vi "WPI_CANJaguar_ScheduleStatusUpdates.vi"(6 "Update Period (s)":dbl=0.1, 8 "error in (no error)":errorcluster, 9 "Status Channel Select":T1, 10 "Status Select":T2[](array[typedef]), 11 "CAN Jaguar Ref":T3={"DeviceStatus"={"status"=FALSE, "code"=0, "source"=""}, "Type"=enum."PWM", "PWM"={"PWM Channel"=enum."PWM 1", "DeadBand"={"Name"="", "maxPositivePwm"=0, "minPositivePwm"=0, "centerPwm"=0, "maxNegativePwm"=0, "minNegativePwm"=0, "angularRange"=0}}, "CAN"={"Device Number"=0, "SetOutput VI Ref"=variant(enum8{"Percent VBus", "Current", "Speed", "Position", "Voltage"} enum."Percent VBus"), "GetOutput VI Ref"=variant(refnum<k1> refnum), "Enable VI Ref"=variant(dbl 12.0), "Disable VI Ref"=variant(enum8{"Percent VBus", "Speed", "Position", "Slave", "Unchanged / Invalid", "Voltage Compensation", "Current", "Motion Profile"} enum."Percent VBus"), "Data"=variant}, "Invert"=FALSE}) -> (0 "error out":errorcluster, 3 "CAN Jaguar Ref Out":T3={"DeviceStatus"={"status"=FALSE, "code"=0, "source"=""}, "Type"=enum."PWM", "PWM"={"PWM Channel"=enum."PWM 1", "DeadBand"={"Name"="", "maxPositivePwm"=0, "minPositivePwm"=0, "centerPwm"=0, "maxNegativePwm"=0, "minNegativePwm"=0, "angularRange"=0}}, "CAN"={"Device Number"=0, "SetOutput VI Ref"=variant(enum8{"Percent VBus", "Current", "Speed", "Position", "Voltage"} enum."Percent VBus"), "GetOutput VI Ref"=variant(refnum<k1> refnum), "Enable VI Ref"=variant(dbl 12.0), "Disable VI Ref"=variant(enum8{"Percent VBus", "Speed", "Position", "Slave", "Unchanged / Invalid", "Voltage Compensation", "Current", "Motion Profile"} enum."Percent VBus"), "Data"=variant}, "Invert"=FALSE})   [LabVIEW 2016]
doc: "Schedule periodic status updates from a CAN Jaguar.\n\nThis VI allows you to specify which parts of the status you care about and how often you want to be updated. If used appropriately, this could reduce the bandwidth needed to get status by more than 50% because the request message is not sent for each update and multiple status values are packaged into a single message.\n\nThe periodic status messages can return 8 bytes of status data on each channel. Be sure that the status messages you select for each channel add up to 8 bytes or less. Output Voltage, Bus Voltage, Current, and Temperature are 2 bytes each. Position and Speed are 4 bytes each. Limit Switches and Faults are 1 byte each. Fault Counters are 8 bytes. Power Cycle is not supported.\n\nSticky Limit Switches, Faults, and Fault Counters are cleared by reading the respective status by calling <B>Get Status</B> VI with <B>Status Channel Select</B> set to <B>On Demand</B>.\n\nWire an empty <B>Status Select</B> array to disable periodic status updates for the channel.\n\nCall the <B>Get Status</B> VI with matching <B>Status Channel Select</B> to read the most recent values sent by the Jaguar."
uses:
  <vilib>/Rock Robotics/WPI/MotorControl/WPI_MotorControlDeviceRef.ctl
  <vilib>/Rock Robotics/WPI/MotorControl/WPI_MotorControlType.ctl
  <vilib>/Rock Robotics/SystemInterfaces/DIO/FPGA_DIOPWMChannel.ctl
  <vilib>/Rock Robotics/WPI/PWM/WPI_PWMDeadband.ctl
  <vilib>/Rock Robotics/WPI/ThirdParty/CanMotor/CAN Jaguar/SubVIs/WPI_CANJaguar_StatusSelect.ctl
  <vilib>/Rock Robotics/WPI/ThirdParty/CanMotor/CAN Jaguar/SubVIs/WPI_CANJaguar_StatusChannelSelect.ctl
  <vilib>/Rock Robotics/WPI/ThirdParty/CanMotor/CAN Jaguar/SubVIs/WPI_CAN_PeriodicStatusIDs.ctl
  <vilib>/Rock Robotics/WPI/ThirdParty/CanMotor/CAN Jaguar/SubVIs/WPI_CAN_MotorMessageIDs.ctl
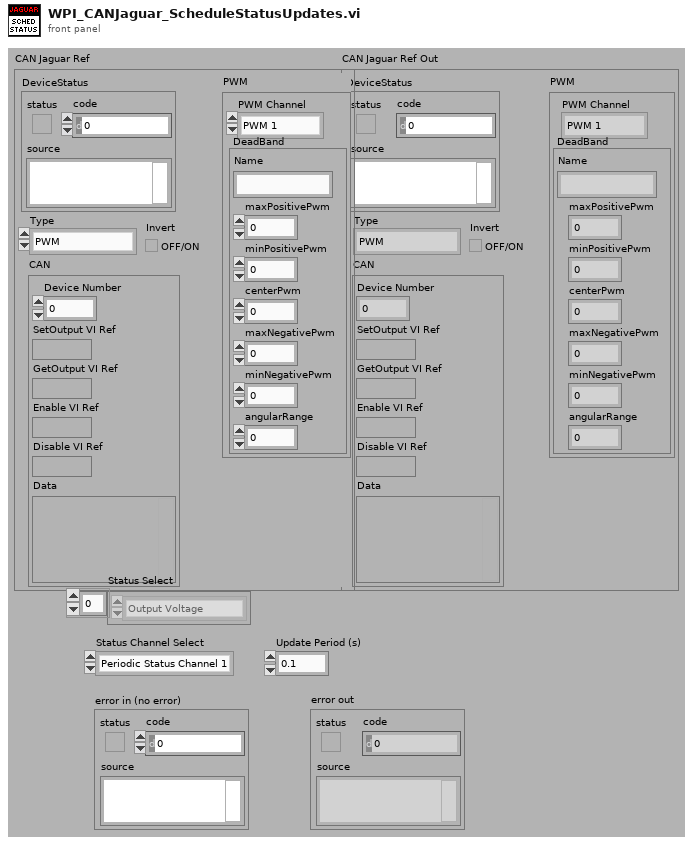
[diagram p1: front panel]
types:
  T1 = typedef "WPI_CANJaguar_StatusChannelSelect.ctl" = enum16{"Periodic Status Channel 1", "Periodic Status Channel 2", "Periodic Status Channel 3", "Periodic Status Channel 4", "On Demand Status"}
  T2 = typedef "WPI_CANJaguar_StatusSelect.ctl" = enum16{"Output Percent VBus", "Output Voltage", "Bus Voltage", "Current", "Temperature", "Position", "Speed", "Limit Switches", "Faults", "Fault Counters", "Power Cycle"}
  T3 = typedef "WPI_MotorControlDeviceRef.ctl" = cluster{"DeviceStatus":errorcluster, "Type":T4, "PWM":cluster{"PWM Channel":T5, "DeadBand":T6}, "CAN":cluster{"Device Number":u8, "SetOutput VI Ref":variant, "GetOutput VI Ref":variant, "Enable VI Ref":variant, "Disable VI Ref":variant, "Data":variant}, "Invert":bool}
  T4 = typedef "WPI_MotorControlType.ctl" = enum16{"PWM", "CAN"}
  T5 = typedef "FPGA_DIOPWMChannel.ctl" = enum8{"PWM 0", "PWM 1", "PWM 2", "PWM 3", "PWM 4", "PWM 5", "PWM 6", "PWM 7", "PWM 8", "PWM 9", "PWM MXP 0", "PWM MXP 1", "PWM MXP 2", "PWM MXP 3", "PWM MXP 4", "PWM MXP 5", "PWM MXP 6", "PWM MXP 7", "PWM MXP 8", "PWM MXP 9", "Invalid"}
  T6 = typedef "WPI_PWMDeadband.ctl" = cluster{"Name":string, "maxPositivePwm":i32, "minPositivePwm":i32, "centerPwm":i32, "maxNegativePwm":i32, "minNegativePwm":i32, "angularRange":u16}
  T7 = typedef "WPI_CAN_PeriodicStatusIDs.ctl" = enum16{"Disabled", "Percent VBus Out (Byte 0)", "Percent VBus Out (Byte 1)", "VBus (Byte 0)", "VBus (Byte 1)", "Current (Byte 0)", "Current (Byte 1)", "Temperature (Byte 0)", "Temperature (Byte 1)", "Position (Byte 0)", "Position (Byte 1)", "Position (Byte 2)", "Position (Byte 3)", "Speed (Byte 0)", "Speed (Byte 1)", "Speed (Byte 2)", "Speed (Byte 3)", "Limit Switches (No Clear)", "Limit Switches (Clear)", "Faults", "Sticky Faults (No Clear)", "Sticky Faults (Clear)", "Volts Out (Byte 0)", "Volts Out (Byte 1)", "Current Fault Counter", "Temperature Fault Counter", "VBus Fault Counter", "Gate Driver Fault Counter", "Comm Fault Counter", "CANSTS", "CANERR (Byte 0)", "CANERR (Byte 1)", "Power Cycle"}
  T8 = enum16{"big-endian, network order", "native, host order", "little-endian"}
  T9 = typedef "WPI_CAN_MotorMessageIDs.ctl" = u32
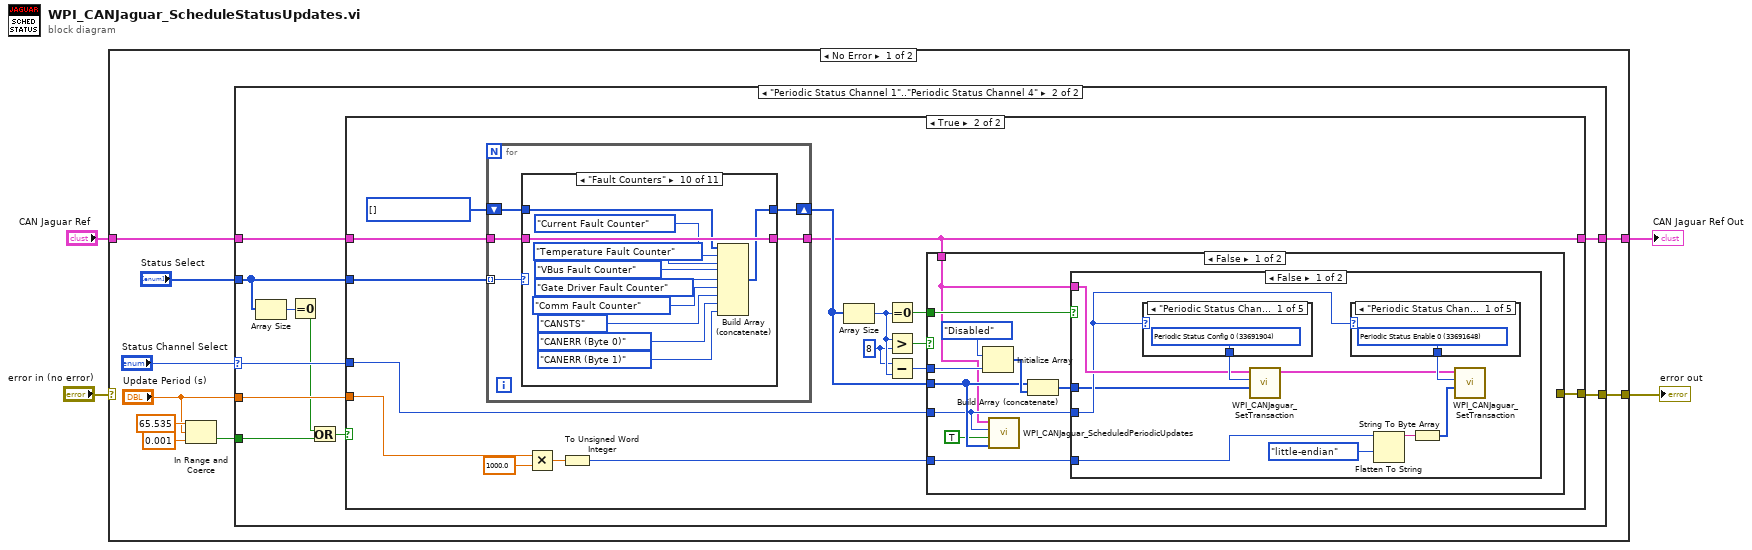
[diagram p0: block diagram]
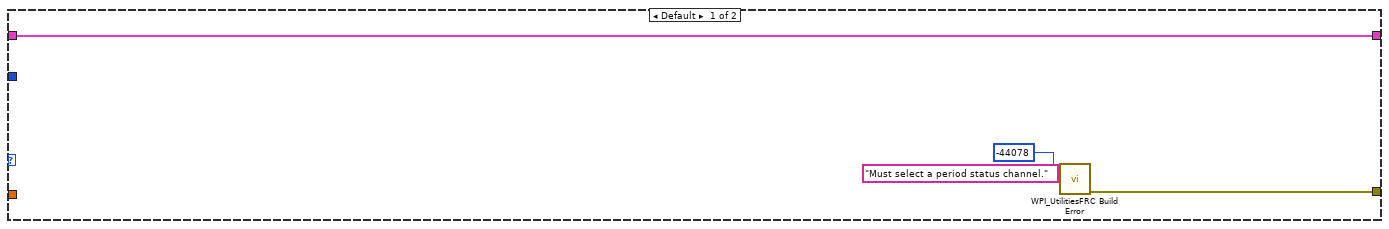
[diagram p2: hidden frame]
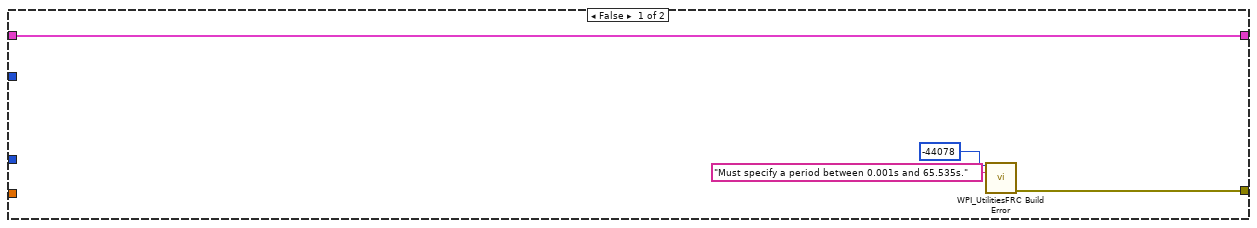
[diagram p3: hidden frame]
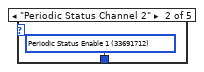
[diagram p4: hidden frame]
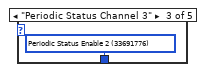
[diagram p5: hidden frame]
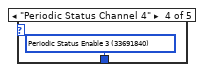
[diagram p6: hidden frame]
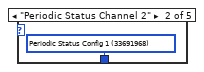
[diagram p8: hidden frame]
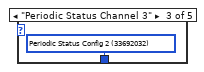
[diagram p9: hidden frame]
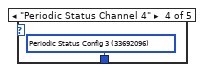
[diagram p10: hidden frame]
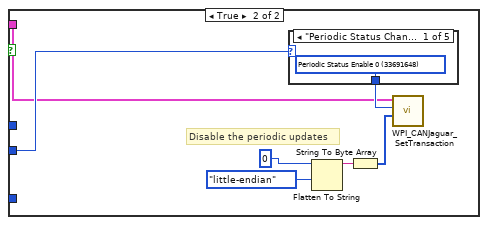
[diagram p12: hidden frame]
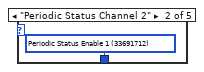
[diagram p13: hidden frame]
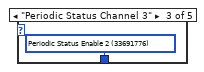
[diagram p14: hidden frame]
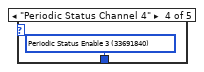
[diagram p15: hidden frame]
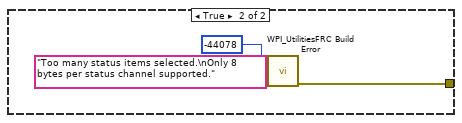
[diagram p17: hidden frame]
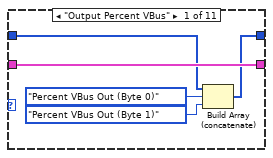
[diagram p18: hidden frame]
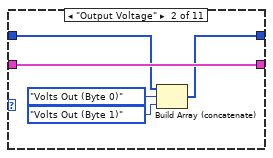
[diagram p19: hidden frame]
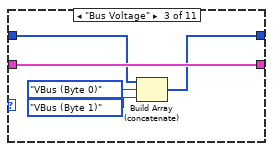
[diagram p20: hidden frame]
diagram:
  n1 = case shown="No Error" "error in (no error)" {
    selector: "error in (no error)" -> [_ w156]
    tunnel: [w11 w155] -> w4
    tunnel: "CAN Jaguar Ref" -> [w13 w155]
    tunnel: [w12 w156] -> w2
    frame No Error {
      n2 = In Range and Coerce(upper limit=65.535, x="Update Period (s)", lower limit=0.001) -> (In Range?=w9:bool)  [unwired: 1 out]
      n3 = case shown="\"Periodic Status Channel 1\"..\"Periodic Status Channel 4\"" "Status Channel Select" {
        selector: "Status Channel Select" -> [_ w24]
        tunnel: w13 -> [w14 w27]
        tunnel: [w15 w26] -> w12
        tunnel: [w14 w25] -> w11
        tunnel: w9 -> [_ w20]
        tunnel: "Update Period (s)" -> [_ w23]
        tunnel: "Status Select" -> [_ w21]
        frame Default {
          n4 = call <vilib>:"WPI_UtilitiesFRC Build Error.vi"("error code"=-44078, "extra error text"="Must select a period status channel.") -> ("error out"=w15:errorcluster)  [unwired: 3 in, 10 out]
        }
        frame "Periodic Status Channel 1".."Periodic Status Channel 4" {
          n5 = Array Size(array=w21) -> (size(s)=w22:i32)
          n6 = Equal To 0?(x=w22) -> (x = 0?=w18:bool)
          n7 = Or(x=w18, y=w20) -> (x .or. y?=w19:bool)
          n8 = case shown="True" w19 {
            tunnel: w27 -> [w28 w47]
            tunnel: [w29 w44] -> w26
            tunnel: [w28 w42] -> w25
            tunnel: w24 -> [_ w41]
            tunnel: w23 -> [_ w40]
            tunnel: w21 -> [_ w32]
            frame False {
              n9 = call <vilib>:"WPI_UtilitiesFRC Build Error.vi"("error code"=-44078, "extra error text"="Must specify a period between 0.001s and 65.535s.") -> ("error out"=w29:errorcluster)  [unwired: 3 in, 10 out]
            }
            frame True {
              w34 = 8 ("y")
              w46 = T7[] [] items=["Disabled", "Percent VBus Out (Byte 0)", "Percent VBus Out (Byte 1)", "VBus (Byte 0)", "VBus (Byte 1)", "Current (Byte 0)", "Current (Byte 1)", "Temperature (Byte 0)", "Temperature (Byte 1)", "Position (Byte 0)", "Position (Byte 1)", "Position (Byte 2)", "Position (Byte 3)", "Speed (Byte 0)", "Speed (Byte 1)", "Speed (Byte 2)", "Speed (Byte 3)", "Limit Switches (No Clear)", "Limit Switches (Clear)", "Faults", "Sticky Faults (No Clear)", "Sticky Faults (Clear)", "Volts Out (Byte 0)", "Volts Out (Byte 1)", "Current Fault Counter", "Temperature Fault Counter", "VBus Fault Counter", "Gate Driver Fault Counter", "Comm Fault Counter", "CANSTS", "CANERR (Byte 0)", "CANERR (Byte 1)", "Power Cycle"]
              n10 = for {
                tunnel: w32 -> [w94] mode=indexing
                tunnel: w47 -> [w93]
                tunnel: [w92] -> w42
                shift-right: [w90] -> w43
                shift-left: w46 -> [w91]
                n11 = case shown="\"Fault Counters\"" w94 {
                  tunnel: w93 -> [w99 w104 w109 w114 w119 w126 w133 w137 w141 w152 w154]
                  tunnel: [w99 w104 w109 w114 w119 w126 w133 w137 w141 w152 w154] -> w92
                  tunnel: w91 -> [w98 w103 w108 w113 w118 w125 w131 w136 w140 w151 w153]
                  tunnel: [w97 w102 w105 w112 w117 w124 w130 w135 w139 w150 w153] -> w90
                  frame "Output Percent VBus" {
                    n12 = Build Array (concatenate)(w98, WPI_CAN_PeriodicStatusIDs."Percent VBus Out (Byte 0)" ("Periodic Status IDs"), WPI_CAN_PeriodicStatusIDs."Percent VBus Out (Byte 1)" ("Periodic Status IDs")) -> (w97:T7[])
                  }
                  frame "Output Voltage" {
                    n13 = Build Array (concatenate)(w103, WPI_CAN_PeriodicStatusIDs."Volts Out (Byte 0)" ("Periodic Status IDs"), WPI_CAN_PeriodicStatusIDs."Volts Out (Byte 1)" ("Periodic Status IDs")) -> (w102:T7[])
                  }
                  frame "Bus Voltage" {
                    n14 = Build Array (concatenate)(w108, WPI_CAN_PeriodicStatusIDs."VBus (Byte 0)" ("Periodic Status IDs"), WPI_CAN_PeriodicStatusIDs."VBus (Byte 1)" ("Periodic Status IDs")) -> (w105:T7[])
                  }
                  frame "Current" {
                    n15 = Build Array (concatenate)(w113, WPI_CAN_PeriodicStatusIDs."Current (Byte 0)" ("Periodic Status IDs"), WPI_CAN_PeriodicStatusIDs."Current (Byte 1)" ("Periodic Status IDs")) -> (w112:T7[])
                  }
                  frame "Temperature" {
                    n16 = Build Array (concatenate)(w118, WPI_CAN_PeriodicStatusIDs."Temperature (Byte 0)" ("Periodic Status IDs"), WPI_CAN_PeriodicStatusIDs."Temperature (Byte 1)" ("Periodic Status IDs")) -> (w117:T7[])
                  }
                  frame "Position" {
                    n17 = Build Array (concatenate)(w125, WPI_CAN_PeriodicStatusIDs."Position (Byte 0)" ("Periodic Status IDs"), WPI_CAN_PeriodicStatusIDs."Position (Byte 1)" ("Periodic Status IDs"), WPI_CAN_PeriodicStatusIDs."Position (Byte 2)" ("Periodic Status IDs"), WPI_CAN_PeriodicStatusIDs."Position (Byte 3)" ("Periodic Status IDs")) -> (w124:T7[])
                  }
                  frame "Speed" {
                    n18 = Build Array (concatenate)(w131, WPI_CAN_PeriodicStatusIDs."Speed (Byte 0)" ("Periodic Status IDs"), WPI_CAN_PeriodicStatusIDs."Speed (Byte 1)" ("Periodic Status IDs"), WPI_CAN_PeriodicStatusIDs."Speed (Byte 2)" ("Periodic Status IDs"), WPI_CAN_PeriodicStatusIDs."Speed (Byte 3)" ("Periodic Status IDs")) -> (w130:T7[])
                  }
                  frame "Limit Switches" {
                    n19 = Build Array (concatenate)(w136, WPI_CAN_PeriodicStatusIDs."Limit Switches (No Clear)" ("Periodic Status IDs")) -> (w135:T7[])
                  }
                  frame "Faults" {
                    n20 = Build Array (concatenate)(w140, WPI_CAN_PeriodicStatusIDs."Sticky Faults (No Clear)" ("Periodic Status IDs")) -> (w139:T7[])
                  }
                  frame "Fault Counters" {
                    n21 = Build Array (concatenate)(w151, WPI_CAN_PeriodicStatusIDs."Current Fault Counter" ("Periodic Status IDs"), WPI_CAN_PeriodicStatusIDs."Temperature Fault Counter" ("Periodic Status IDs"), WPI_CAN_PeriodicStatusIDs."VBus Fault Counter" ("Periodic Status IDs"), WPI_CAN_PeriodicStatusIDs."Gate Driver Fault Counter" ("Periodic Status IDs"), WPI_CAN_PeriodicStatusIDs."Comm Fault Counter" ("Periodic Status IDs"), WPI_CAN_PeriodicStatusIDs."CANSTS" ("Periodic Status IDs"), WPI_CAN_PeriodicStatusIDs."CANERR (Byte 0)" ("Periodic Status IDs"), WPI_CAN_PeriodicStatusIDs."CANERR (Byte 1)" ("Periodic Status IDs")) -> (w150:T7[])
                  }
                  frame "Power Cycle" {
                  }
                }
              }
              n22 = Multiply(x=w40, y=1000.0) -> (x*y=w38:dbl)
              n23 = To Unsigned Word Integer(number=w38) -> (unsigned 16bit integer=w37:u16)
              n24 = Array Size(array=w43) -> (size(s)=w35:i32)
              n25 = Equal To 0?(x=w35) -> (x = 0?=w36:bool)
              n26 = Greater?(x=w35, y=w34) -> (0:w45:bool)
              n27 = Subtract(x=w34, y=w35) -> (x-y=w33:i32)
              n28 = case shown="False" w45 {
                tunnel: [_ w87] -> w44
                tunnel: w43 -> [w51 _]
                tunnel: w42 -> [w48 _]
                tunnel: w41 -> [w49 _]
                tunnel: w37 -> [w57 _]
                tunnel: w36 -> [w56 _]
                tunnel: w33 -> [w55 _]
                frame False {
                  n29 = Initialize Array(WPI_CAN_PeriodicStatusIDs."Disabled" ("Periodic Status IDs"), w55) -> (w52:T7[])
                  n30 = call <vilib>:"WPI_CANJaguar_ScheduledPeriodicUpdates.vi"("Fields In"=w51, "Update"=TRUE, "Status Channel Select"=w49, "CAN Jaguar Ref"=w48) -> ()  [unwired: 7 in, 1 out]
                  n31 = Build Array (concatenate)(w51, w52) -> (w53:T7[])
                  n32 = case shown="False" w56 {
                    tunnel: w48 -> [w65 w76]
                    tunnel: w57 -> [w60 _]
                    tunnel: w49 -> [w59 w77]
                    tunnel: w53 -> [w58 _]
                    frame False {
                      n33 = case shown="\"Periodic Status Channel 1\"" w59 {
                        tunnel: [w72 w73 w74 w75 _] -> w67
                        frame "Periodic Status Channel 1" {
                          w72 = T9 33691904 items=["Volt Enable"=33685504, "Volt Disable"=33685568, "Volt Set"=33685632, "Volt Set Ramp"=33685696, "Volt Set No Ack"=33686080, "Speed Enable"=33686528, "Speed Disable"=33686592, "Speed Set"=33686656, "Speed P"=33686720, "Speed I"=33686784, "Speed D"=33686848, "Speed Ref"=33686912, "Speed Set No Ack"=33687232, "Volt Comp Enable"=33687552, "Volt Comp Disable"=33687616, "Volt Comp Set"=33687680, "Volt Comp In Ramp"=33687744, "Volt Comp Comp Ramp"=33687808, "Volt Comp Set No Ack"=33688128, "Position Enable"=33688576, "Position Disable"=33688640, "Position Set"=33688704, "Position P"=33688768, "Position I"=33688832, "Position D"=33688896, "Position Ref"=33688960, "Position Set No Ack"=33689280, "Current Enable"=33689600, "Current Disable"=33689664, "Current Set"=33689728, "Current P"=33689792, "Current I"=33689856, "Current D"=33689920, "Current Set No Ack"=33690240, "Status Percent VBus"=33690624, "Status VBus"=33690688, "Status Current"=33690752, "Status Temp"=33690816, "Status Position"=33690880, "Status Speed"=33690944, "Status Limit"=33691008, "Status Fault"=33691072, "Status Power"=33691136, "Status Control Mode"=33691200, "Status VOut"=33691264, "Status Sticky Fault"=33691328, "Status Fault Count"=33691392, "Periodic Status Enable 0"=33691648, "Periodic Status Enable 1"=33691712, "Periodic Status Enable 2"=33691776, "Periodic Status Enable 3"=33691840, "Periodic Status Config 0"=33691904, "Periodic Status Config 1"=33691968, "Periodic Status Config 2"=33692032, "Periodic Status Config 3"=33692096, "Periodic Status Data 0"=33692160, "Periodic Status Data 1"=33692224, "Periodic Status Data 2"=33692288, "Periodic Status Data 3"=33692352, "Config Num Brushes"=33692672, "Config Encoder Lines"=33692736, "Config Pot Turns"=33692800, "Config Brake Coast"=33692864, "Config Limit Mode"=33692928, "Config Limit Fwd"=33692992, "Config Limit Rev"=33693056, "Config Max VOut"=33693120, "Config Fault Time"=33693184, "Motor Ack"=33693696] ("CAN Motor Message IDs")
                        }
                        frame "Periodic Status Channel 2" {
                          w73 = T9 33691968 items=["Volt Enable"=33685504, "Volt Disable"=33685568, "Volt Set"=33685632, "Volt Set Ramp"=33685696, "Volt Set No Ack"=33686080, "Speed Enable"=33686528, "Speed Disable"=33686592, "Speed Set"=33686656, "Speed P"=33686720, "Speed I"=33686784, "Speed D"=33686848, "Speed Ref"=33686912, "Speed Set No Ack"=33687232, "Volt Comp Enable"=33687552, "Volt Comp Disable"=33687616, "Volt Comp Set"=33687680, "Volt Comp In Ramp"=33687744, "Volt Comp Comp Ramp"=33687808, "Volt Comp Set No Ack"=33688128, "Position Enable"=33688576, "Position Disable"=33688640, "Position Set"=33688704, "Position P"=33688768, "Position I"=33688832, "Position D"=33688896, "Position Ref"=33688960, "Position Set No Ack"=33689280, "Current Enable"=33689600, "Current Disable"=33689664, "Current Set"=33689728, "Current P"=33689792, "Current I"=33689856, "Current D"=33689920, "Current Set No Ack"=33690240, "Status Percent VBus"=33690624, "Status VBus"=33690688, "Status Current"=33690752, "Status Temp"=33690816, "Status Position"=33690880, "Status Speed"=33690944, "Status Limit"=33691008, "Status Fault"=33691072, "Status Power"=33691136, "Status Control Mode"=33691200, "Status VOut"=33691264, "Status Sticky Fault"=33691328, "Status Fault Count"=33691392, "Periodic Status Enable 0"=33691648, "Periodic Status Enable 1"=33691712, "Periodic Status Enable 2"=33691776, "Periodic Status Enable 3"=33691840, "Periodic Status Config 0"=33691904, "Periodic Status Config 1"=33691968, "Periodic Status Config 2"=33692032, "Periodic Status Config 3"=33692096, "Periodic Status Data 0"=33692160, "Periodic Status Data 1"=33692224, "Periodic Status Data 2"=33692288, "Periodic Status Data 3"=33692352, "Config Num Brushes"=33692672, "Config Encoder Lines"=33692736, "Config Pot Turns"=33692800, "Config Brake Coast"=33692864, "Config Limit Mode"=33692928, "Config Limit Fwd"=33692992, "Config Limit Rev"=33693056, "Config Max VOut"=33693120, "Config Fault Time"=33693184, "Motor Ack"=33693696] ("CAN Motor Message IDs")
                        }
                        frame "Periodic Status Channel 3" {
                          w74 = T9 33692032 items=["Volt Enable"=33685504, "Volt Disable"=33685568, "Volt Set"=33685632, "Volt Set Ramp"=33685696, "Volt Set No Ack"=33686080, "Speed Enable"=33686528, "Speed Disable"=33686592, "Speed Set"=33686656, "Speed P"=33686720, "Speed I"=33686784, "Speed D"=33686848, "Speed Ref"=33686912, "Speed Set No Ack"=33687232, "Volt Comp Enable"=33687552, "Volt Comp Disable"=33687616, "Volt Comp Set"=33687680, "Volt Comp In Ramp"=33687744, "Volt Comp Comp Ramp"=33687808, "Volt Comp Set No Ack"=33688128, "Position Enable"=33688576, "Position Disable"=33688640, "Position Set"=33688704, "Position P"=33688768, "Position I"=33688832, "Position D"=33688896, "Position Ref"=33688960, "Position Set No Ack"=33689280, "Current Enable"=33689600, "Current Disable"=33689664, "Current Set"=33689728, "Current P"=33689792, "Current I"=33689856, "Current D"=33689920, "Current Set No Ack"=33690240, "Status Percent VBus"=33690624, "Status VBus"=33690688, "Status Current"=33690752, "Status Temp"=33690816, "Status Position"=33690880, "Status Speed"=33690944, "Status Limit"=33691008, "Status Fault"=33691072, "Status Power"=33691136, "Status Control Mode"=33691200, "Status VOut"=33691264, "Status Sticky Fault"=33691328, "Status Fault Count"=33691392, "Periodic Status Enable 0"=33691648, "Periodic Status Enable 1"=33691712, "Periodic Status Enable 2"=33691776, "Periodic Status Enable 3"=33691840, "Periodic Status Config 0"=33691904, "Periodic Status Config 1"=33691968, "Periodic Status Config 2"=33692032, "Periodic Status Config 3"=33692096, "Periodic Status Data 0"=33692160, "Periodic Status Data 1"=33692224, "Periodic Status Data 2"=33692288, "Periodic Status Data 3"=33692352, "Config Num Brushes"=33692672, "Config Encoder Lines"=33692736, "Config Pot Turns"=33692800, "Config Brake Coast"=33692864, "Config Limit Mode"=33692928, "Config Limit Fwd"=33692992, "Config Limit Rev"=33693056, "Config Max VOut"=33693120, "Config Fault Time"=33693184, "Motor Ack"=33693696] ("CAN Motor Message IDs")
                        }
                        frame "Periodic Status Channel 4" {
                          w75 = T9 33692096 items=["Volt Enable"=33685504, "Volt Disable"=33685568, "Volt Set"=33685632, "Volt Set Ramp"=33685696, "Volt Set No Ack"=33686080, "Speed Enable"=33686528, "Speed Disable"=33686592, "Speed Set"=33686656, "Speed P"=33686720, "Speed I"=33686784, "Speed D"=33686848, "Speed Ref"=33686912, "Speed Set No Ack"=33687232, "Volt Comp Enable"=33687552, "Volt Comp Disable"=33687616, "Volt Comp Set"=33687680, "Volt Comp In Ramp"=33687744, "Volt Comp Comp Ramp"=33687808, "Volt Comp Set No Ack"=33688128, "Position Enable"=33688576, "Position Disable"=33688640, "Position Set"=33688704, "Position P"=33688768, "Position I"=33688832, "Position D"=33688896, "Position Ref"=33688960, "Position Set No Ack"=33689280, "Current Enable"=33689600, "Current Disable"=33689664, "Current Set"=33689728, "Current P"=33689792, "Current I"=33689856, "Current D"=33689920, "Current Set No Ack"=33690240, "Status Percent VBus"=33690624, "Status VBus"=33690688, "Status Current"=33690752, "Status Temp"=33690816, "Status Position"=33690880, "Status Speed"=33690944, "Status Limit"=33691008, "Status Fault"=33691072, "Status Power"=33691136, "Status Control Mode"=33691200, "Status VOut"=33691264, "Status Sticky Fault"=33691328, "Status Fault Count"=33691392, "Periodic Status Enable 0"=33691648, "Periodic Status Enable 1"=33691712, "Periodic Status Enable 2"=33691776, "Periodic Status Enable 3"=33691840, "Periodic Status Config 0"=33691904, "Periodic Status Config 1"=33691968, "Periodic Status Config 2"=33692032, "Periodic Status Config 3"=33692096, "Periodic Status Data 0"=33692160, "Periodic Status Data 1"=33692224, "Periodic Status Data 2"=33692288, "Periodic Status Data 3"=33692352, "Config Num Brushes"=33692672, "Config Encoder Lines"=33692736, "Config Pot Turns"=33692800, "Config Brake Coast"=33692864, "Config Limit Mode"=33692928, "Config Limit Fwd"=33692992, "Config Limit Rev"=33693056, "Config Max VOut"=33693120, "Config Fault Time"=33693184, "Motor Ack"=33693696] ("CAN Motor Message IDs")
                        }
                        frame Default {
                          # "This won't happen"
                        }
                      }
                      n34 = call <vilib>:"WPI_CANJaguar_SetTransaction.vi"("Data"=w58, "Message ID"=w67, "CAN Jaguar Ref"=w65) -> ("CAN Jaguar Ref Out"=w64:T3)  [unwired: 1 in, 7 out]
                      n35 = case shown="\"Periodic Status Channel 1\"" w59 {
                        tunnel: [w68 w69 w70 w71 _] -> w66
                        frame "Periodic Status Channel 1" {
                          w68 = T9 33691648 items=["Volt Enable"=33685504, "Volt Disable"=33685568, "Volt Set"=33685632, "Volt Set Ramp"=33685696, "Volt Set No Ack"=33686080, "Speed Enable"=33686528, "Speed Disable"=33686592, "Speed Set"=33686656, "Speed P"=33686720, "Speed I"=33686784, "Speed D"=33686848, "Speed Ref"=33686912, "Speed Set No Ack"=33687232, "Volt Comp Enable"=33687552, "Volt Comp Disable"=33687616, "Volt Comp Set"=33687680, "Volt Comp In Ramp"=33687744, "Volt Comp Comp Ramp"=33687808, "Volt Comp Set No Ack"=33688128, "Position Enable"=33688576, "Position Disable"=33688640, "Position Set"=33688704, "Position P"=33688768, "Position I"=33688832, "Position D"=33688896, "Position Ref"=33688960, "Position Set No Ack"=33689280, "Current Enable"=33689600, "Current Disable"=33689664, "Current Set"=33689728, "Current P"=33689792, "Current I"=33689856, "Current D"=33689920, "Current Set No Ack"=33690240, "Status Percent VBus"=33690624, "Status VBus"=33690688, "Status Current"=33690752, "Status Temp"=33690816, "Status Position"=33690880, "Status Speed"=33690944, "Status Limit"=33691008, "Status Fault"=33691072, "Status Power"=33691136, "Status Control Mode"=33691200, "Status VOut"=33691264, "Status Sticky Fault"=33691328, "Status Fault Count"=33691392, "Periodic Status Enable 0"=33691648, "Periodic Status Enable 1"=33691712, "Periodic Status Enable 2"=33691776, "Periodic Status Enable 3"=33691840, "Periodic Status Config 0"=33691904, "Periodic Status Config 1"=33691968, "Periodic Status Config 2"=33692032, "Periodic Status Config 3"=33692096, "Periodic Status Data 0"=33692160, "Periodic Status Data 1"=33692224, "Periodic Status Data 2"=33692288, "Periodic Status Data 3"=33692352, "Config Num Brushes"=33692672, "Config Encoder Lines"=33692736, "Config Pot Turns"=33692800, "Config Brake Coast"=33692864, "Config Limit Mode"=33692928, "Config Limit Fwd"=33692992, "Config Limit Rev"=33693056, "Config Max VOut"=33693120, "Config Fault Time"=33693184, "Motor Ack"=33693696] ("CAN Motor Message IDs")
                        }
                        frame "Periodic Status Channel 2" {
                          w69 = T9 33691712 items=["Volt Enable"=33685504, "Volt Disable"=33685568, "Volt Set"=33685632, "Volt Set Ramp"=33685696, "Volt Set No Ack"=33686080, "Speed Enable"=33686528, "Speed Disable"=33686592, "Speed Set"=33686656, "Speed P"=33686720, "Speed I"=33686784, "Speed D"=33686848, "Speed Ref"=33686912, "Speed Set No Ack"=33687232, "Volt Comp Enable"=33687552, "Volt Comp Disable"=33687616, "Volt Comp Set"=33687680, "Volt Comp In Ramp"=33687744, "Volt Comp Comp Ramp"=33687808, "Volt Comp Set No Ack"=33688128, "Position Enable"=33688576, "Position Disable"=33688640, "Position Set"=33688704, "Position P"=33688768, "Position I"=33688832, "Position D"=33688896, "Position Ref"=33688960, "Position Set No Ack"=33689280, "Current Enable"=33689600, "Current Disable"=33689664, "Current Set"=33689728, "Current P"=33689792, "Current I"=33689856, "Current D"=33689920, "Current Set No Ack"=33690240, "Status Percent VBus"=33690624, "Status VBus"=33690688, "Status Current"=33690752, "Status Temp"=33690816, "Status Position"=33690880, "Status Speed"=33690944, "Status Limit"=33691008, "Status Fault"=33691072, "Status Power"=33691136, "Status Control Mode"=33691200, "Status VOut"=33691264, "Status Sticky Fault"=33691328, "Status Fault Count"=33691392, "Periodic Status Enable 0"=33691648, "Periodic Status Enable 1"=33691712, "Periodic Status Enable 2"=33691776, "Periodic Status Enable 3"=33691840, "Periodic Status Config 0"=33691904, "Periodic Status Config 1"=33691968, "Periodic Status Config 2"=33692032, "Periodic Status Config 3"=33692096, "Periodic Status Data 0"=33692160, "Periodic Status Data 1"=33692224, "Periodic Status Data 2"=33692288, "Periodic Status Data 3"=33692352, "Config Num Brushes"=33692672, "Config Encoder Lines"=33692736, "Config Pot Turns"=33692800, "Config Brake Coast"=33692864, "Config Limit Mode"=33692928, "Config Limit Fwd"=33692992, "Config Limit Rev"=33693056, "Config Max VOut"=33693120, "Config Fault Time"=33693184, "Motor Ack"=33693696] ("CAN Motor Message IDs")
                        }
                        frame "Periodic Status Channel 3" {
                          w70 = T9 33691776 items=["Volt Enable"=33685504, "Volt Disable"=33685568, "Volt Set"=33685632, "Volt Set Ramp"=33685696, "Volt Set No Ack"=33686080, "Speed Enable"=33686528, "Speed Disable"=33686592, "Speed Set"=33686656, "Speed P"=33686720, "Speed I"=33686784, "Speed D"=33686848, "Speed Ref"=33686912, "Speed Set No Ack"=33687232, "Volt Comp Enable"=33687552, "Volt Comp Disable"=33687616, "Volt Comp Set"=33687680, "Volt Comp In Ramp"=33687744, "Volt Comp Comp Ramp"=33687808, "Volt Comp Set No Ack"=33688128, "Position Enable"=33688576, "Position Disable"=33688640, "Position Set"=33688704, "Position P"=33688768, "Position I"=33688832, "Position D"=33688896, "Position Ref"=33688960, "Position Set No Ack"=33689280, "Current Enable"=33689600, "Current Disable"=33689664, "Current Set"=33689728, "Current P"=33689792, "Current I"=33689856, "Current D"=33689920, "Current Set No Ack"=33690240, "Status Percent VBus"=33690624, "Status VBus"=33690688, "Status Current"=33690752, "Status Temp"=33690816, "Status Position"=33690880, "Status Speed"=33690944, "Status Limit"=33691008, "Status Fault"=33691072, "Status Power"=33691136, "Status Control Mode"=33691200, "Status VOut"=33691264, "Status Sticky Fault"=33691328, "Status Fault Count"=33691392, "Periodic Status Enable 0"=33691648, "Periodic Status Enable 1"=33691712, "Periodic Status Enable 2"=33691776, "Periodic Status Enable 3"=33691840, "Periodic Status Config 0"=33691904, "Periodic Status Config 1"=33691968, "Periodic Status Config 2"=33692032, "Periodic Status Config 3"=33692096, "Periodic Status Data 0"=33692160, "Periodic Status Data 1"=33692224, "Periodic Status Data 2"=33692288, "Periodic Status Data 3"=33692352, "Config Num Brushes"=33692672, "Config Encoder Lines"=33692736, "Config Pot Turns"=33692800, "Config Brake Coast"=33692864, "Config Limit Mode"=33692928, "Config Limit Fwd"=33692992, "Config Limit Rev"=33693056, "Config Max VOut"=33693120, "Config Fault Time"=33693184, "Motor Ack"=33693696] ("CAN Motor Message IDs")
                        }
                        frame "Periodic Status Channel 4" {
                          w71 = T9 33691840 items=["Volt Enable"=33685504, "Volt Disable"=33685568, "Volt Set"=33685632, "Volt Set Ramp"=33685696, "Volt Set No Ack"=33686080, "Speed Enable"=33686528, "Speed Disable"=33686592, "Speed Set"=33686656, "Speed P"=33686720, "Speed I"=33686784, "Speed D"=33686848, "Speed Ref"=33686912, "Speed Set No Ack"=33687232, "Volt Comp Enable"=33687552, "Volt Comp Disable"=33687616, "Volt Comp Set"=33687680, "Volt Comp In Ramp"=33687744, "Volt Comp Comp Ramp"=33687808, "Volt Comp Set No Ack"=33688128, "Position Enable"=33688576, "Position Disable"=33688640, "Position Set"=33688704, "Position P"=33688768, "Position I"=33688832, "Position D"=33688896, "Position Ref"=33688960, "Position Set No Ack"=33689280, "Current Enable"=33689600, "Current Disable"=33689664, "Current Set"=33689728, "Current P"=33689792, "Current I"=33689856, "Current D"=33689920, "Current Set No Ack"=33690240, "Status Percent VBus"=33690624, "Status VBus"=33690688, "Status Current"=33690752, "Status Temp"=33690816, "Status Position"=33690880, "Status Speed"=33690944, "Status Limit"=33691008, "Status Fault"=33691072, "Status Power"=33691136, "Status Control Mode"=33691200, "Status VOut"=33691264, "Status Sticky Fault"=33691328, "Status Fault Count"=33691392, "Periodic Status Enable 0"=33691648, "Periodic Status Enable 1"=33691712, "Periodic Status Enable 2"=33691776, "Periodic Status Enable 3"=33691840, "Periodic Status Config 0"=33691904, "Periodic Status Config 1"=33691968, "Periodic Status Config 2"=33692032, "Periodic Status Config 3"=33692096, "Periodic Status Data 0"=33692160, "Periodic Status Data 1"=33692224, "Periodic Status Data 2"=33692288, "Periodic Status Data 3"=33692352, "Config Num Brushes"=33692672, "Config Encoder Lines"=33692736, "Config Pot Turns"=33692800, "Config Brake Coast"=33692864, "Config Limit Mode"=33692928, "Config Limit Fwd"=33692992, "Config Limit Rev"=33693056, "Config Max VOut"=33693120, "Config Fault Time"=33693184, "Motor Ack"=33693696] ("CAN Motor Message IDs")
                        }
                        frame Default {
                          # "This won't happen"
                        }
                      }
                      n36 = Flatten To String(anything=w60, byte order (0:big-endian, network order)=T8."little-endian") -> (data string=w62:string)  [unwired: 1 in, 3 out]
                      n37 = String To Byte Array(string=w62) -> (unsigned byte array=w61:u8[])
                      n38 = call <vilib>:"WPI_CANJaguar_SetTransaction.vi"("Data"=w61, "Message ID"=w66, "CAN Jaguar Ref"=w64) -> ()  [unwired: 1 in, 8 out]
                    }
                    frame True {
                      # "Disable the periodic updates"
                      n39 = case shown="\"Periodic Status Channel 1\"" w77 {
                        tunnel: [w83 w84 w85 w86 _] -> w82
                        frame "Periodic Status Channel 1" {
                          w83 = T9 33691648 items=["Volt Enable"=33685504, "Volt Disable"=33685568, "Volt Set"=33685632, "Volt Set Ramp"=33685696, "Volt Set No Ack"=33686080, "Speed Enable"=33686528, "Speed Disable"=33686592, "Speed Set"=33686656, "Speed P"=33686720, "Speed I"=33686784, "Speed D"=33686848, "Speed Ref"=33686912, "Speed Set No Ack"=33687232, "Volt Comp Enable"=33687552, "Volt Comp Disable"=33687616, "Volt Comp Set"=33687680, "Volt Comp In Ramp"=33687744, "Volt Comp Comp Ramp"=33687808, "Volt Comp Set No Ack"=33688128, "Position Enable"=33688576, "Position Disable"=33688640, "Position Set"=33688704, "Position P"=33688768, "Position I"=33688832, "Position D"=33688896, "Position Ref"=33688960, "Position Set No Ack"=33689280, "Current Enable"=33689600, "Current Disable"=33689664, "Current Set"=33689728, "Current P"=33689792, "Current I"=33689856, "Current D"=33689920, "Current Set No Ack"=33690240, "Status Percent VBus"=33690624, "Status VBus"=33690688, "Status Current"=33690752, "Status Temp"=33690816, "Status Position"=33690880, "Status Speed"=33690944, "Status Limit"=33691008, "Status Fault"=33691072, "Status Power"=33691136, "Status Control Mode"=33691200, "Status VOut"=33691264, "Status Sticky Fault"=33691328, "Status Fault Count"=33691392, "Periodic Status Enable 0"=33691648, "Periodic Status Enable 1"=33691712, "Periodic Status Enable 2"=33691776, "Periodic Status Enable 3"=33691840, "Periodic Status Config 0"=33691904, "Periodic Status Config 1"=33691968, "Periodic Status Config 2"=33692032, "Periodic Status Config 3"=33692096, "Periodic Status Data 0"=33692160, "Periodic Status Data 1"=33692224, "Periodic Status Data 2"=33692288, "Periodic Status Data 3"=33692352, "Config Num Brushes"=33692672, "Config Encoder Lines"=33692736, "Config Pot Turns"=33692800, "Config Brake Coast"=33692864, "Config Limit Mode"=33692928, "Config Limit Fwd"=33692992, "Config Limit Rev"=33693056, "Config Max VOut"=33693120, "Config Fault Time"=33693184, "Motor Ack"=33693696] ("CAN Motor Message IDs")
                        }
                        frame "Periodic Status Channel 2" {
                          w84 = T9 33691712 items=["Volt Enable"=33685504, "Volt Disable"=33685568, "Volt Set"=33685632, "Volt Set Ramp"=33685696, "Volt Set No Ack"=33686080, "Speed Enable"=33686528, "Speed Disable"=33686592, "Speed Set"=33686656, "Speed P"=33686720, "Speed I"=33686784, "Speed D"=33686848, "Speed Ref"=33686912, "Speed Set No Ack"=33687232, "Volt Comp Enable"=33687552, "Volt Comp Disable"=33687616, "Volt Comp Set"=33687680, "Volt Comp In Ramp"=33687744, "Volt Comp Comp Ramp"=33687808, "Volt Comp Set No Ack"=33688128, "Position Enable"=33688576, "Position Disable"=33688640, "Position Set"=33688704, "Position P"=33688768, "Position I"=33688832, "Position D"=33688896, "Position Ref"=33688960, "Position Set No Ack"=33689280, "Current Enable"=33689600, "Current Disable"=33689664, "Current Set"=33689728, "Current P"=33689792, "Current I"=33689856, "Current D"=33689920, "Current Set No Ack"=33690240, "Status Percent VBus"=33690624, "Status VBus"=33690688, "Status Current"=33690752, "Status Temp"=33690816, "Status Position"=33690880, "Status Speed"=33690944, "Status Limit"=33691008, "Status Fault"=33691072, "Status Power"=33691136, "Status Control Mode"=33691200, "Status VOut"=33691264, "Status Sticky Fault"=33691328, "Status Fault Count"=33691392, "Periodic Status Enable 0"=33691648, "Periodic Status Enable 1"=33691712, "Periodic Status Enable 2"=33691776, "Periodic Status Enable 3"=33691840, "Periodic Status Config 0"=33691904, "Periodic Status Config 1"=33691968, "Periodic Status Config 2"=33692032, "Periodic Status Config 3"=33692096, "Periodic Status Data 0"=33692160, "Periodic Status Data 1"=33692224, "Periodic Status Data 2"=33692288, "Periodic Status Data 3"=33692352, "Config Num Brushes"=33692672, "Config Encoder Lines"=33692736, "Config Pot Turns"=33692800, "Config Brake Coast"=33692864, "Config Limit Mode"=33692928, "Config Limit Fwd"=33692992, "Config Limit Rev"=33693056, "Config Max VOut"=33693120, "Config Fault Time"=33693184, "Motor Ack"=33693696] ("CAN Motor Message IDs")
                        }
                        frame "Periodic Status Channel 3" {
                          w85 = T9 33691776 items=["Volt Enable"=33685504, "Volt Disable"=33685568, "Volt Set"=33685632, "Volt Set Ramp"=33685696, "Volt Set No Ack"=33686080, "Speed Enable"=33686528, "Speed Disable"=33686592, "Speed Set"=33686656, "Speed P"=33686720, "Speed I"=33686784, "Speed D"=33686848, "Speed Ref"=33686912, "Speed Set No Ack"=33687232, "Volt Comp Enable"=33687552, "Volt Comp Disable"=33687616, "Volt Comp Set"=33687680, "Volt Comp In Ramp"=33687744, "Volt Comp Comp Ramp"=33687808, "Volt Comp Set No Ack"=33688128, "Position Enable"=33688576, "Position Disable"=33688640, "Position Set"=33688704, "Position P"=33688768, "Position I"=33688832, "Position D"=33688896, "Position Ref"=33688960, "Position Set No Ack"=33689280, "Current Enable"=33689600, "Current Disable"=33689664, "Current Set"=33689728, "Current P"=33689792, "Current I"=33689856, "Current D"=33689920, "Current Set No Ack"=33690240, "Status Percent VBus"=33690624, "Status VBus"=33690688, "Status Current"=33690752, "Status Temp"=33690816, "Status Position"=33690880, "Status Speed"=33690944, "Status Limit"=33691008, "Status Fault"=33691072, "Status Power"=33691136, "Status Control Mode"=33691200, "Status VOut"=33691264, "Status Sticky Fault"=33691328, "Status Fault Count"=33691392, "Periodic Status Enable 0"=33691648, "Periodic Status Enable 1"=33691712, "Periodic Status Enable 2"=33691776, "Periodic Status Enable 3"=33691840, "Periodic Status Config 0"=33691904, "Periodic Status Config 1"=33691968, "Periodic Status Config 2"=33692032, "Periodic Status Config 3"=33692096, "Periodic Status Data 0"=33692160, "Periodic Status Data 1"=33692224, "Periodic Status Data 2"=33692288, "Periodic Status Data 3"=33692352, "Config Num Brushes"=33692672, "Config Encoder Lines"=33692736, "Config Pot Turns"=33692800, "Config Brake Coast"=33692864, "Config Limit Mode"=33692928, "Config Limit Fwd"=33692992, "Config Limit Rev"=33693056, "Config Max VOut"=33693120, "Config Fault Time"=33693184, "Motor Ack"=33693696] ("CAN Motor Message IDs")
                        }
                        frame "Periodic Status Channel 4" {
                          w86 = T9 33691840 items=["Volt Enable"=33685504, "Volt Disable"=33685568, "Volt Set"=33685632, "Volt Set Ramp"=33685696, "Volt Set No Ack"=33686080, "Speed Enable"=33686528, "Speed Disable"=33686592, "Speed Set"=33686656, "Speed P"=33686720, "Speed I"=33686784, "Speed D"=33686848, "Speed Ref"=33686912, "Speed Set No Ack"=33687232, "Volt Comp Enable"=33687552, "Volt Comp Disable"=33687616, "Volt Comp Set"=33687680, "Volt Comp In Ramp"=33687744, "Volt Comp Comp Ramp"=33687808, "Volt Comp Set No Ack"=33688128, "Position Enable"=33688576, "Position Disable"=33688640, "Position Set"=33688704, "Position P"=33688768, "Position I"=33688832, "Position D"=33688896, "Position Ref"=33688960, "Position Set No Ack"=33689280, "Current Enable"=33689600, "Current Disable"=33689664, "Current Set"=33689728, "Current P"=33689792, "Current I"=33689856, "Current D"=33689920, "Current Set No Ack"=33690240, "Status Percent VBus"=33690624, "Status VBus"=33690688, "Status Current"=33690752, "Status Temp"=33690816, "Status Position"=33690880, "Status Speed"=33690944, "Status Limit"=33691008, "Status Fault"=33691072, "Status Power"=33691136, "Status Control Mode"=33691200, "Status VOut"=33691264, "Status Sticky Fault"=33691328, "Status Fault Count"=33691392, "Periodic Status Enable 0"=33691648, "Periodic Status Enable 1"=33691712, "Periodic Status Enable 2"=33691776, "Periodic Status Enable 3"=33691840, "Periodic Status Config 0"=33691904, "Periodic Status Config 1"=33691968, "Periodic Status Config 2"=33692032, "Periodic Status Config 3"=33692096, "Periodic Status Data 0"=33692160, "Periodic Status Data 1"=33692224, "Periodic Status Data 2"=33692288, "Periodic Status Data 3"=33692352, "Config Num Brushes"=33692672, "Config Encoder Lines"=33692736, "Config Pot Turns"=33692800, "Config Brake Coast"=33692864, "Config Limit Mode"=33692928, "Config Limit Fwd"=33692992, "Config Limit Rev"=33693056, "Config Max VOut"=33693120, "Config Fault Time"=33693184, "Motor Ack"=33693696] ("CAN Motor Message IDs")
                        }
                        frame Default {
                          # "This won't happen"
                        }
                      }
                      n40 = Flatten To String(anything=u16 0, byte order (0:big-endian, network order)=T8."little-endian") -> (data string=w80:string)  [unwired: 1 in, 3 out]
                      n41 = String To Byte Array(string=w80) -> (unsigned byte array=w79:u8[])
                      n42 = call <vilib>:"WPI_CANJaguar_SetTransaction.vi"("Data"=w79, "Message ID"=w82, "CAN Jaguar Ref"=w76) -> ()  [unwired: 1 in, 8 out]
                    }
                  }
                }
                frame True {
                  n43 = call <vilib>:"WPI_UtilitiesFRC Build Error.vi"("error code"=-44078, "extra error text"="Too many status items selected.\nOnly 8 bytes per status channel supported.") -> ("error out"=w87:errorcluster)  [unwired: 3 in, 10 out]
                }
              }
            }
          }
        }
      }
    }
    frame Error {
    }
  }
  "CAN Jaguar Ref Out" <- w4
  "error out" <- w2
